vi "Autonomous Independent.vi"() -> ()   [LabVIEW 2013]
doc: "This VI is called when autonomous begins, and will automatically be terminated when autonomous ends. You can carry out timed or sensor driven robot movement independently without needing to return to the caller."
uses:
  <vilib>/Rock Robotics/WPI/Solenoid/WPI_SolenoidValue.ctl
  Robot Global Data.vi
  <vilib>/Rock Robotics/WPI/Solenoid/WPI_SolenoidSetEnum.vi
  <vilib>/Rock Robotics/WPI/RobotDrive/WPI_RobotDriveGetSetRefNum.vi
panel:
  in  "Velocidade direita":dbl=0.69 format="%#_13g"
  in  "Velocidade esquerda":dbl=0.7
  in  "Tempo(s)":dbl=4.0 format="%#_13g"
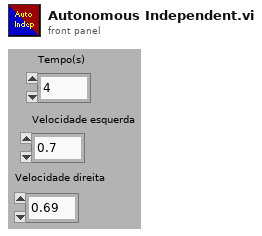
[diagram p1: front panel]
types:
  T1 = enum16{"START", "ONE", "TWO ", "TREE", "FOUR", "FIVE"}
  T2 = typedef "WPI_DigitalInputDevRef.ctl" = cluster{"DevStatus":errorcluster, "DIO Channel":T3, "Digital Module":T4}
  T3 = typedef "FPGA_DIOChannel.ctl" = enum8{"DIO 1", "DIO 2", "DIO 3", "DIO 4", "DIO 5", "DIO 6", "DIO 7", "DIO 8", "DIO 9", "DIO 10", "DIO 11", "DIO 12", "DIO 13", "DIO 14", "Invalid"}
  T4 = typedef "FPGA_TypedefDigitalModule.ctl" = enum16{"Digital Module 1", "Digital Module 2"}
  T5 = typedef "WPI_MotorControlDeviceRef.ctl" = cluster{"DeviceStatus":errorcluster, "Type":enum16{"PWM", "CAN"}, "PWM":cluster{"Digital Module":T4, "PWM Channel":T6, "DeadBand":T7}, "CAN":cluster{"Device Number":u8, "Control Mode":T8, "Semaphore":T9, "Max Vout":dbl}, "Invert":bool, "TransformRef":T10, "InvTransformRef":T10}
  T6 = typedef "FPGA_DIOPWMChannel.ctl" = enum8{"PWM 1", "PWM 2", "PWM 3", "PWM 4", "PWM 5", "PWM 6", "PWM 7", "PWM 8", "PWM 9", "PWM 10", "Invalid"}
  T7 = typedef "WPI_PWMDeadband.ctl" = cluster{"Name":string, "maxPositivePwm":i32, "minPositivePwm":i32, "centerPwm":i32, "maxNegativePwm":i32, "minNegativePwm":i32, "angularRange":u16}
  T8 = typedef "WPI_CANJaguar_ControlMode.ctl" = enum8{"Percent VBus", "Current", "Speed", "Position", "Voltage"}
  T9 = typedef "Semaphore RefNum" = refnum<k1>
  T10 = typedef "WPI_PWMTransform_ConPane.ctl" = refnum<vi>
  T11 = typedef "WPI_SolenoidValue.ctl" = enum16{"Off", "On", "Forward", "Reverse"}
  T12 = typedef "WPI_SolenoidDevRef.ctl" = cluster{"DevStatus":errorcluster, "Solenoid Module":T13, "Forward Solenoid Channel":T14, "Reverse Solenoid Channel":T14}
  T13 = typedef "FPGA_TypedefSolenoidModule.ctl" = enum16{"Solenoid Module 1", "Solenoid Module 2"}
  T14 = typedef "WPI_SolenoidChannel.ctl" = enum8{"Solenoid 1", "Solenoid 2", "Solenoid 3", "Solenoid 4", "Solenoid 5", "Solenoid 6", "Solenoid 7", "Solenoid 8", "Invalid"}
  T15 = typedef "WPI_RobotDriveDevRef.ctl" = cluster{"DevStatus":errorcluster, "Motors[]":T5[], "Square Inputs":bool, "Max Output":dbl, "Isochronous":bool}
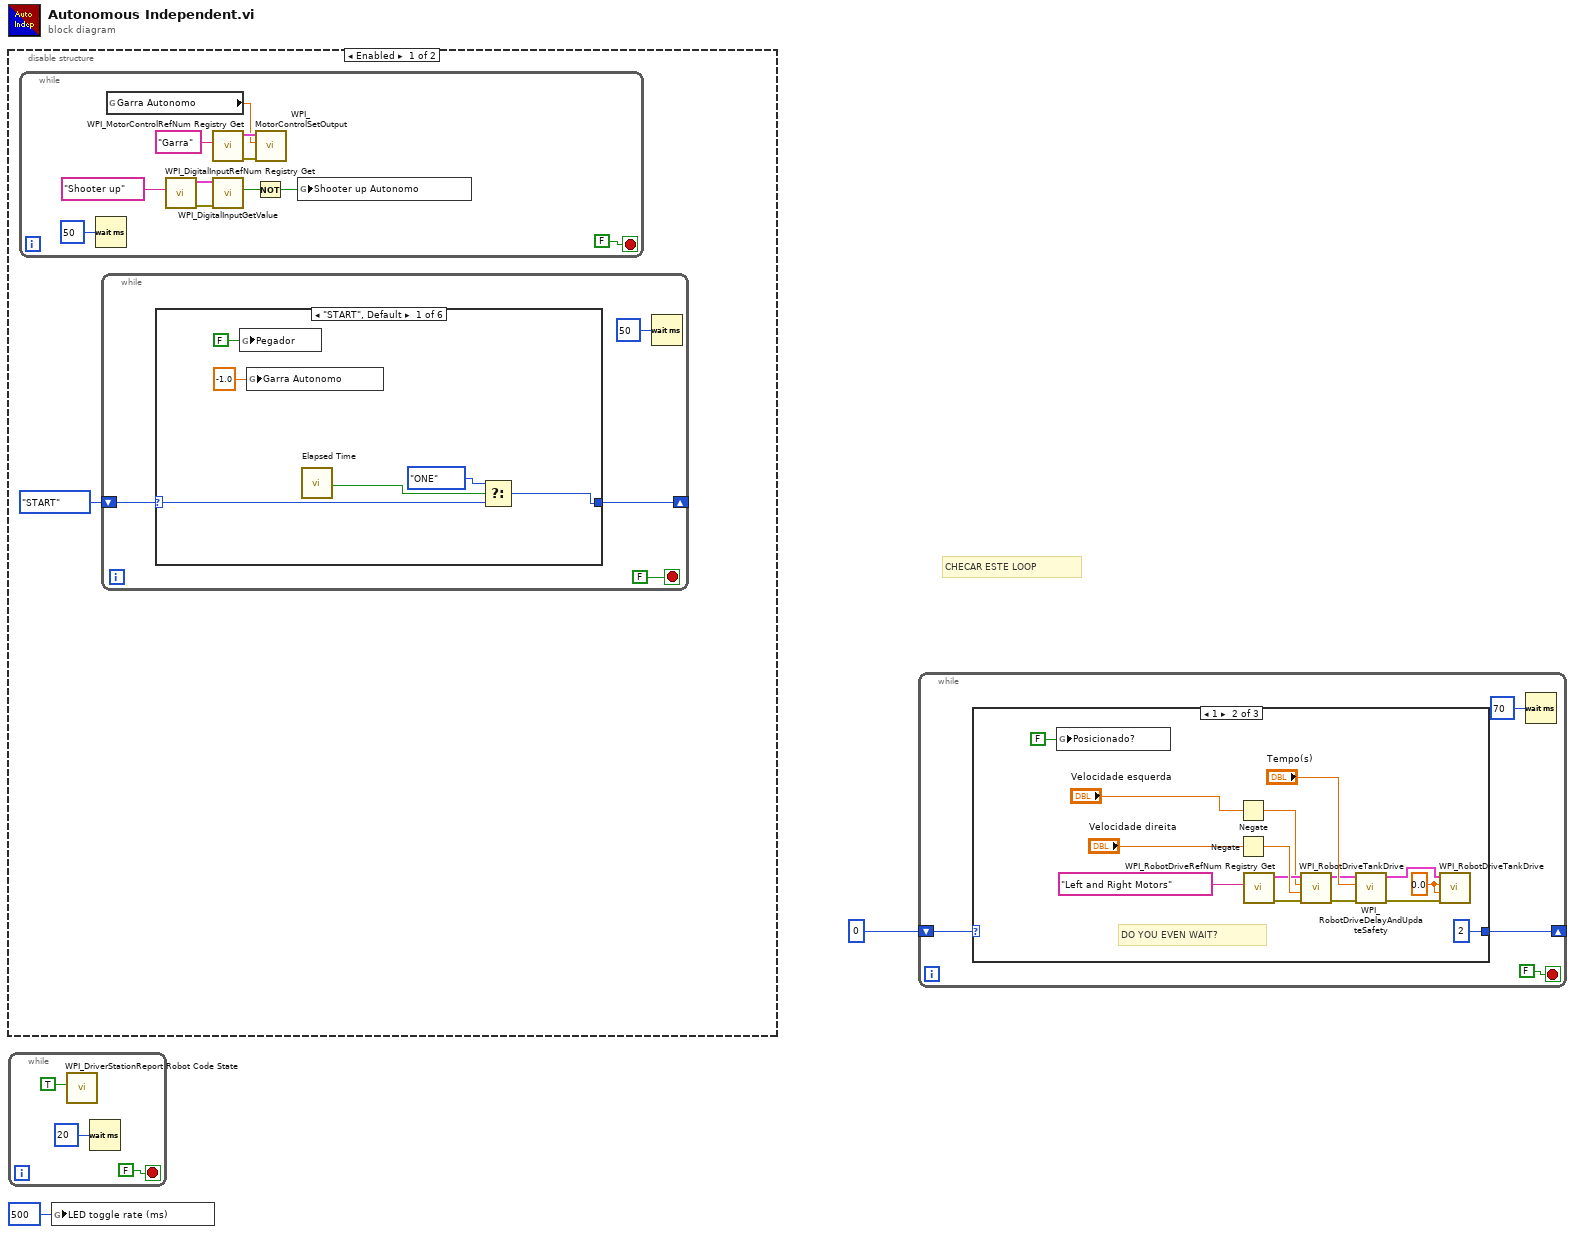
[diagram p0: block diagram]
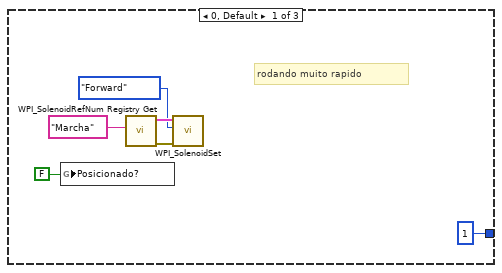
[diagram p2: hidden frame]
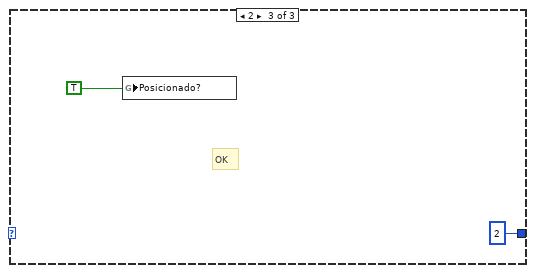
[diagram p3: hidden frame]
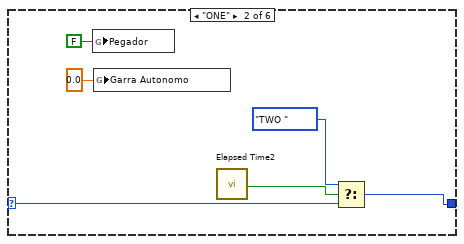
[diagram p4: hidden frame]
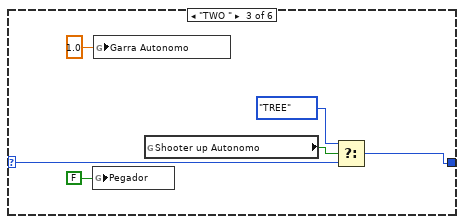
[diagram p5: hidden frame]
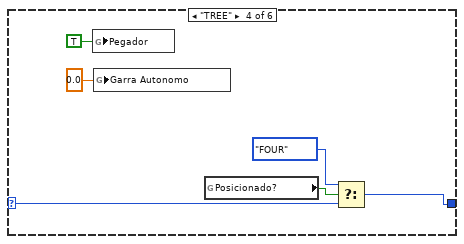
[diagram p6: hidden frame]
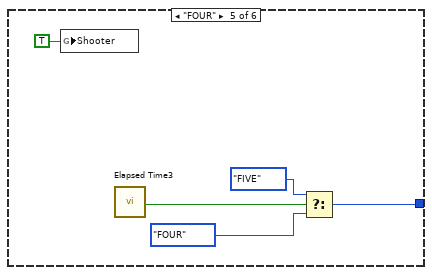
[diagram p7: hidden frame]
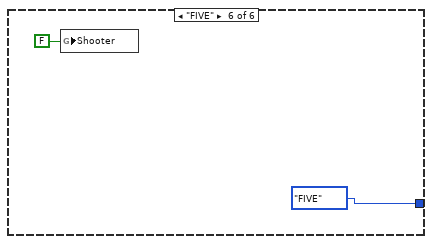
[diagram p8: hidden frame]
diagram:
  # "CHECAR ESTE LOOP"
  n1 = disable-structure shown="Enabled" {
    frame Enabled {
      n2 = while {
        stop <- FALSE stop-if-true
        n3 = Wait (ms)(milliseconds to wait=u32 50) -> ()  [unwired: 1 out]
        n4 = global read "Robot Global Data.vi" "Garra Autonomo"() -> (w5:dbl)
        n5 = call <vilib>:"WPI_DigitalInputRefNum Registry Get.vi"("refnum name"="Shooter up") -> ("error out"=w10:errorcluster, "DigitalInputDevRef"=w9:T2)  [unwired: 9 in]
        n6 = call <vilib>:"WPI_MotorControlRefNum Registry Get.vi"("refnum name"="Garra") -> ("error out"=w12:errorcluster, "MotorControlDevRef"=w13:T5)  [unwired: 9 in]
        n7 = call <vilib>:"WPI_DigitalInputGetValue.vi"("error in (no error)"=w10, "DigitalInputDevRef"=w9) -> ("Value"=w8:bool)  [unwired: 7 in, 2 out]
        n8 = Not(x=w8) -> (.not. x?=w6:bool)
        n9 = call <vilib>:"WPI_MotorControlSetOutput.vi"("error in (no error)"=w12, "Output"=w5, "MotorControlDevRef"=w13) -> ()  [unwired: 6 in, 3 out]
        n10 = global write "Robot Global Data.vi" "Shooter up Autonomo"(w6) -> ()
      }
      n11 = while {
        shift-right: [w17] -> _
        shift-left: T1."START" -> [w18]
        stop <- FALSE stop-if-true
        n12 = case shown="\"START\", Default" w18 {
          selector: w18 -> [w21 w29 w34 w39 _ _]
          tunnel: [w24 w30 w36 w41 w46 T1."FIVE"] -> w17
          frame "START", Default {
            n13 = global write "Robot Global Data.vi" "Pegador"(FALSE ("Pegador")) -> ()
            n14 = global write "Robot Global Data.vi" "Garra Autonomo"(-1.0 ("Garra Autonomo")) -> ()
            n15 = call "Elapsed Time"() -> ("Time has Elapsed"=w22:bool)  [unwired: 12 in, 7 out]
            n16 = Select(t=T1."ONE", s=w22, f=w21) -> (s? t:f=w24:T1)
          }
          frame "ONE" {
            n17 = global write "Robot Global Data.vi" "Pegador"(FALSE ("Pegador")) -> ()
            n18 = global write "Robot Global Data.vi" "Garra Autonomo"(0.0 ("Garra Autonomo")) -> ()
            n19 = call "Elapsed Time2"() -> ("Time has Elapsed"=w27:bool)  [unwired: 12 in, 7 out]
            n20 = Select(t=T1."TWO ", s=w27, f=w29) -> (s? t:f=w30:T1)
          }
          frame "TWO " {
            n21 = global write "Robot Global Data.vi" "Pegador"(FALSE ("Pegador")) -> ()
            n22 = global write "Robot Global Data.vi" "Garra Autonomo"(1.0 ("Garra Autonomo")) -> ()
            n23 = global read "Robot Global Data.vi" "Shooter up Autonomo"() -> (w31:bool)
            n24 = Select(t=T1."TREE", s=w31, f=w34) -> (s? t:f=w36:T1)
          }
          frame "TREE" {
            n25 = global write "Robot Global Data.vi" "Pegador"(TRUE ("Pegador")) -> ()
            n26 = global write "Robot Global Data.vi" "Garra Autonomo"(0.0 ("Garra Autonomo")) -> ()
            n27 = global read "Robot Global Data.vi" "Posicionado?"() -> (w37:bool)
            n28 = Select(t=T1."FOUR", s=w37, f=w39) -> (s? t:f=w41:T1)
          }
          frame "FOUR" {
            n29 = global write "Robot Global Data.vi" "Shooter"(TRUE ("Shooter")) -> ()
            n30 = call "Elapsed Time3"() -> ("Time has Elapsed"=w43:bool)  [unwired: 12 in, 7 out]
            n31 = Select(t=T1."FIVE", s=w43, f=T1."FOUR") -> (s? t:f=w46:T1)
          }
          frame "FIVE" {
            n32 = global write "Robot Global Data.vi" "Shooter"(FALSE ("Shooter")) -> ()
          }
        }
        n33 = Wait (ms)(milliseconds to wait=u32 50) -> ()  [unwired: 1 out]
      }
    }
    frame Disabled {
    }
  }
  n34 = while {
    stop <- FALSE stop-if-true
    n35 = call <vilib>:"WPI_DriverStationReport Robot Code State.vi"("Autonomous"=TRUE) -> ()  [unwired: 10 in, 1 out]
    n36 = Wait (ms)(milliseconds to wait=u32 20) -> ()  [unwired: 1 out]
  }
  n37 = global write "Robot Global Data.vi" "LED toggle rate (ms)"(u32 500 ("LED ms toggle rate")) -> ()
  n38 = while {
    shift-right: [w55] -> _
    shift-left: 0 -> [w56]
    stop <- FALSE stop-if-true
    n39 = case shown="1" w56 {
      tunnel: [1 2 2] -> w55
      frame 0, Default {
        # "rodando muito rapido"
        n40 = global write "Robot Global Data.vi" "Posicionado?"(FALSE ("Posicionado?")) -> ()
        n41 = call <vilib>:"WPI_SolenoidRefNum Registry Get.vi"("refnum name"="Marcha") -> ("error out"=w61:errorcluster, "SolenoidDevRef"=w60:T12)  [unwired: 9 in]
        n42 = call-poly <vilib>:"WPI_SolenoidSet.vi"("error in (no error)"=w61, "Value"=WPI_SolenoidValue."Forward", "SolenoidDevRef"=w60) -> ()  [unwired: 7 in, 2 out]
      }
      frame 1 {
        w76 = 0.0 ("Right axis value")
        # "DO YOU EVEN WAIT?"
        n43 = global write "Robot Global Data.vi" "Posicionado?"(FALSE ("Posicionado?")) -> ()
        n44 = Negate(x="Velocidade esquerda") -> (-x=w66:dbl)
        n45 = Negate(x="Velocidade direita") -> (-x=w77:dbl)
        n46 = call <vilib>:"WPI_RobotDriveRefNum Registry Get.vi"("refnum name"="Left and Right Motors") -> ("error out"=w70:errorcluster, "RobotDriveDevRef"=w69:T15)  [unwired: 9 in]
        n47 = call <vilib>:"WPI_RobotDriveTankDrive.vi"("error in (no error)"=w70, "Right axis value"=w77, "Left axis value"=w66, "RobotDriveDevRef"=w69) -> ("error out"=w72:errorcluster, "RobotDriveDevRef"=w71:T15)  [unwired: 5 in, 1 out]
        n48 = call <vilib>:"WPI_RobotDriveDelayAndUpdateSafety.vi"("error in (no error)"=w72, "Delay (s)"="Tempo(s)", "RobotDriveDevRef"=w71) -> ("error out"=w74:errorcluster, "RobotDriveDevRef 2"=w73:T15)  [unwired: 7 in]
        n49 = call <vilib>:"WPI_RobotDriveTankDrive.vi"("error in (no error)"=w74, "Right axis value"=w76, "Left axis value"=w76, "RobotDriveDevRef"=w73) -> ()  [unwired: 5 in, 3 out]
      }
      frame 2 {
        # "OK"
        n50 = global write "Robot Global Data.vi" "Posicionado?"(TRUE ("Posicionado?")) -> ()
      }
    }
    n51 = Wait (ms)(milliseconds to wait=u32 70) -> ()  [unwired: 1 out]
  }
